vi "Receive Messages Blocking.vi"(8 "error in":errorcluster, 9 "Timeout":i32=1000 format="%d ms", 10 "Sender":string, 11 "Simulated CANopen Node in":refnum<class "Simulated CANopen Node.lvclass">) -> (0 "error out":errorcluster, 1 "Timed out":bool, 2 "IMessages":refnum<class "IMessage.lvclass">[](array[class]), 3 "Simulated CANopen Node out":refnum<class "Simulated CANopen Node.lvclass">)   [LabVIEW 2020, in "Simulated CANopen Node.lvclass"]
uses:
  HAL/Source/Interfaces/IMessage/IMessage.lvclass
  Simulated CANopen Node.lvclass
  Simulated CANopen Node.lvclass/Simulated CANopen Node.ctl
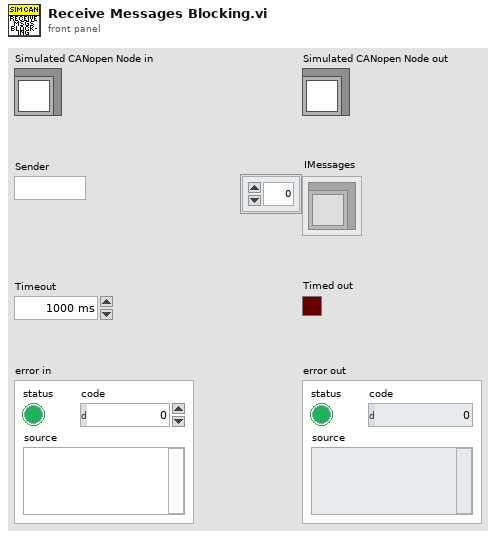
[diagram p1: front panel]
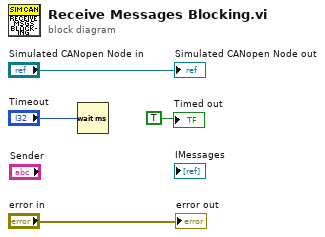
[diagram p0: block diagram]
diagram:
  n1 = Wait (ms)(milliseconds to wait="Timeout") -> ()  [unwired: 1 out]
  "Simulated CANopen Node out" <- "Simulated CANopen Node in"
  "error out" <- "error in"
  "Timed out" <- TRUE ("Timed out")
